vi "Write Component Export Dir.vi"(8 "error in (no error)":errorcluster, 10 "Built Export's Location":path, 11 "Export in":refnum<class "Export.lvclass">) -> (0 "error out":errorcluster, 3 "Export out":refnum<class "Export.lvclass">)   [LabVIEW 2017, in "CL_G3_VIComponentBuilder.lvlib" / "Export.lvclass"]
uses:
  Export.lvclass
  Export.lvclass/Export.ctl
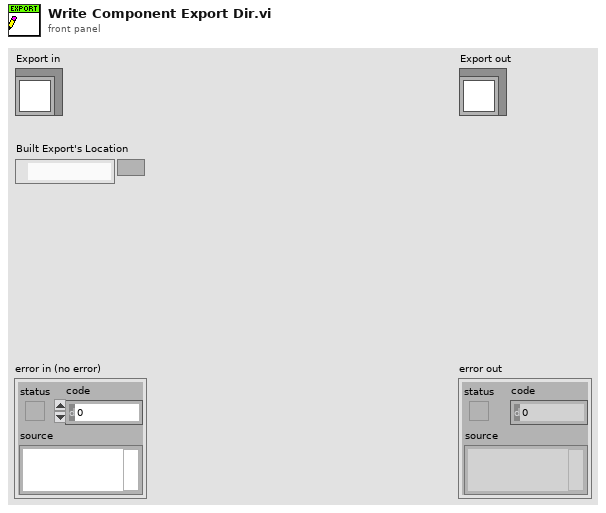
[diagram p1: front panel]
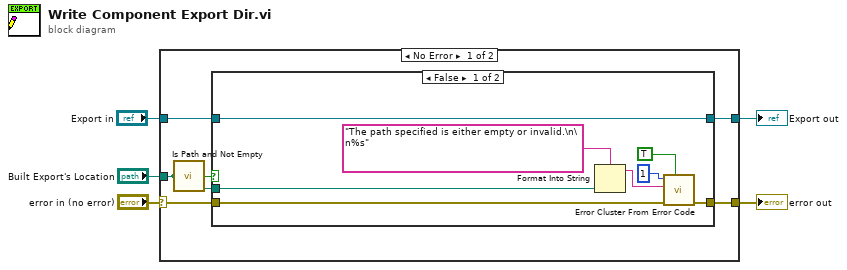
[diagram p0: block diagram]
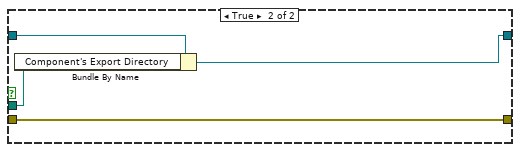
[diagram p2: hidden frame]
diagram:
  n1 = case shown="No Error" "error in (no error)" {
    selector: "error in (no error)" -> [w7 w24]
    tunnel: [w6 w24] -> w4
    tunnel: [w10 w25] -> w2
    tunnel: "Export in" -> [w11 w25]
    tunnel: "Built Export's Location" -> [w9 _]
    frame No Error {
      n2 = call <vilib>:"Is Path and Not Empty.vi"("path"=w9) -> ("Is Path and Not Empty?"=w8:bool)  [unwired: 4 in]
      n3 = case shown="False" w8 {
        tunnel: w11 -> [w12 w23]
        tunnel: [w12 w22] -> w10
        tunnel: w9 -> [w15 w21]
        tunnel: w7 -> [w19 w20]
        tunnel: [w13 w20] -> w6
        frame False {
          n4 = Format Into String(format string="The path specified is either empty or invalid.\n\n%s", w15) -> (resulting string=w14:string)  [unwired: 2 in, 1 out]
          n5 = call <vilib>:"Error Cluster From Error Code.vi"("show call chain? (False)"=TRUE, "error in (no error)"=w19, "error message (\"\")"=w14, "error code (0)"=1) -> ("error out"=w13:errorcluster)  [unwired: 5 in]
        }
        frame True {
          n6 = Bundle By Name(cluster=w23, "Component's Export Directory"=w21) -> (w22:refnum<class "Export.lvclass">)
        }
      }
    }
    frame Error {
    }
  }
  "error out" <- w4
  "Export out" <- w2
